vi "cblas dznrm2.vi"(5 "n":i32=-1, 7 "incx":i32=1, 11 "x":cdb[](array[numeric])) -> (0 "error":i32, 3 "dznrm2":dbl)   [LabVIEW 2018, in "NI_AALBLAS.lvlib"]
uses:
  NI_AALBLAS.lvlib
  <resource>/lvblas.dll
panel:
  # "double cblas_dznrm2(n, *x, incx)"
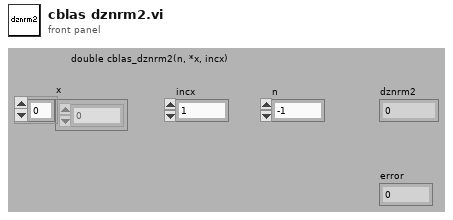
[diagram p1: front panel]
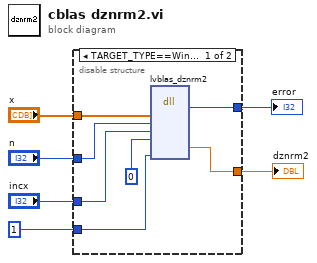
[diagram p0: block diagram]
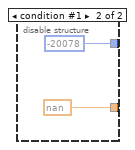
[diagram p2: hidden frame]
diagram:
  n1 = disable-structure shown="TARGET_TYPE==Windows||TARGET_TYPE==Unix||TARGET_TYPE==Mac||TARGET_TYPE==RT" {
    disable-tunnel: "x" -> [w12 _]
    disable-tunnel: "n" -> [w11 _]
    disable-tunnel: "incx" -> [w10 _]
    disable-tunnel: [w8 nan] -> w3
    disable-tunnel: [w13 -20078] -> w2
    disable-tunnel: 1 -> [w7 _]
    frame condition #0 (active) {
      n2 = dll-call lib="C:/Program Files (x86)/National Instruments/LabVIEW 2018/resource/lvblas.*" fn="lvblas_dznrm2" ("LVBLAS.dll:CxBLASVectorNorm2H")("X"=w12, "N"=w11, "IncX"=w10, "startX"=0, "check"=w7) -> ("error"=w13:i32, "norm2"=w8:dbl)  [unwired: 8 in, 3 out]
    }
    frame condition #1 {
    }
  }
  "dznrm2" <- w3
  "error" <- w2
